vi "ProjetaParabola.vi"(11 "file path (dialog if empty)":path=path "adp.csv") -> (0 "Primeiro":dbl[](array[numeric]), 1 "Ultimo":dbl[](array[numeric]))   [LabVIEW 2019]
uses:
  <vilib>/Analysis/coordinate.llb/3D Coordinate Conversion (Array).vi
  <vilib>/Analysis/_algsub.llb/Real Vector Norm.vi
  <vilib>/Utility/file.llb/Read Delimited Spreadsheet (DBL).vi
  <vilib>/Analysis/polynomials.llb/Polynomial Roots (DBL).vi
  <vilib>/Analysis/NI_AALPro.lvlib
  <vilib>/Analysis/NI_AAL_Geometry.lvlib
panel:
  out "chegada":dbl[](array[numeric])
  out "partida":dbl[](array[numeric])
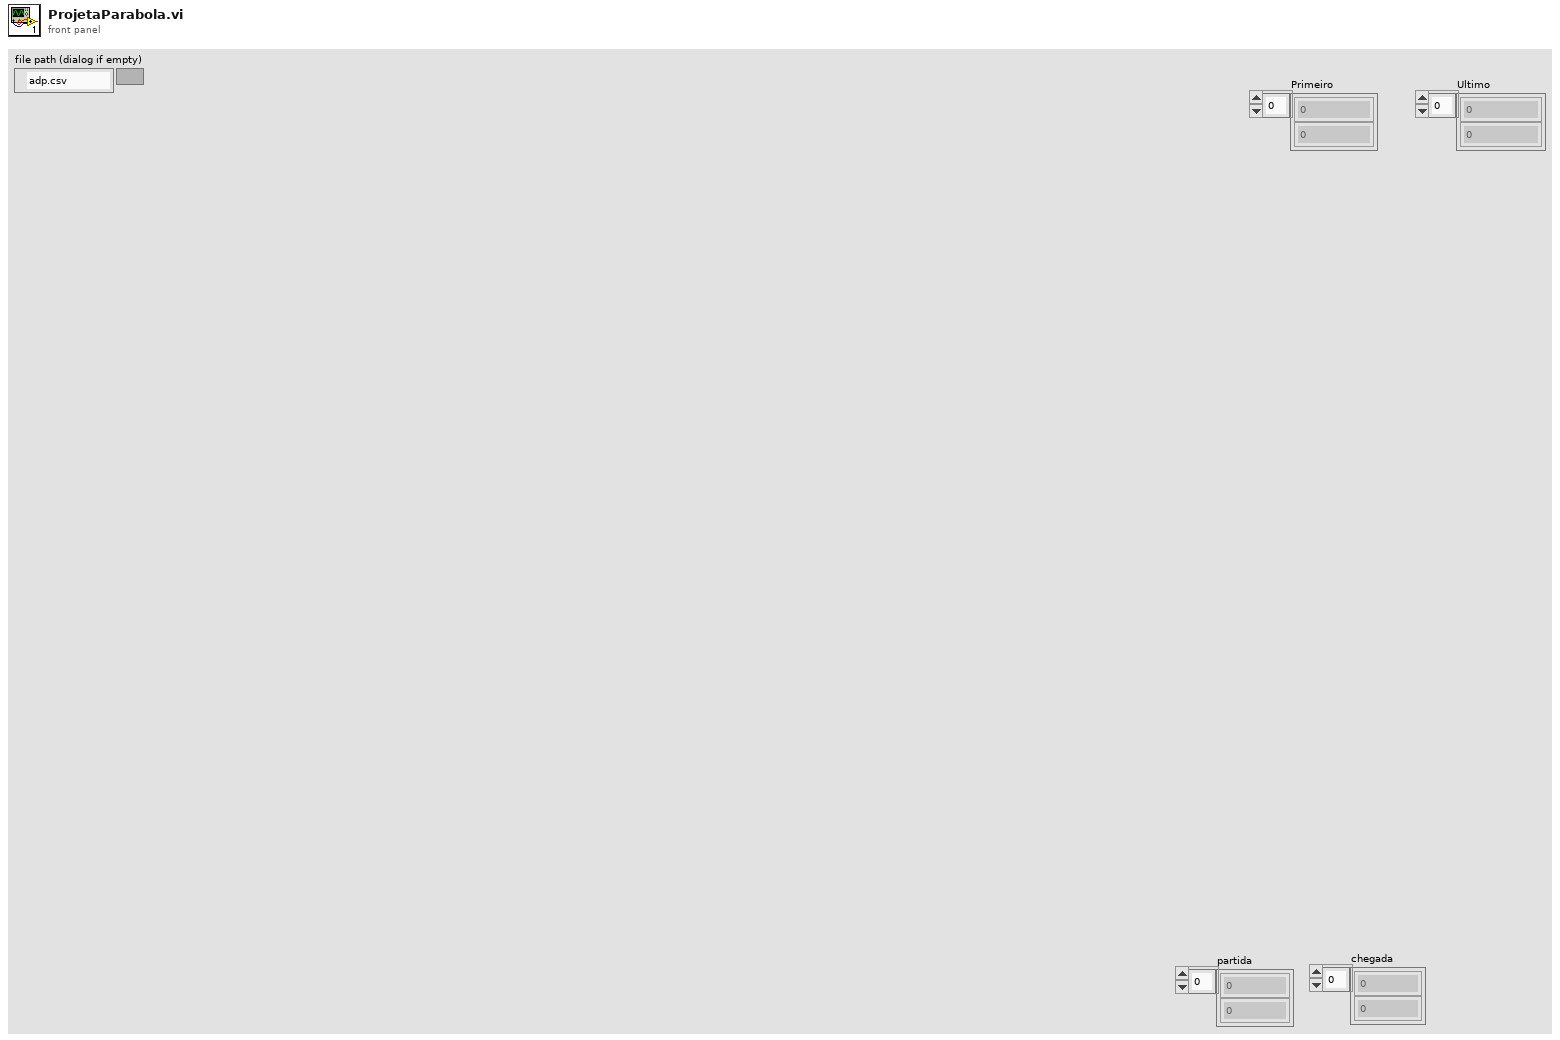
[diagram p1: front panel]
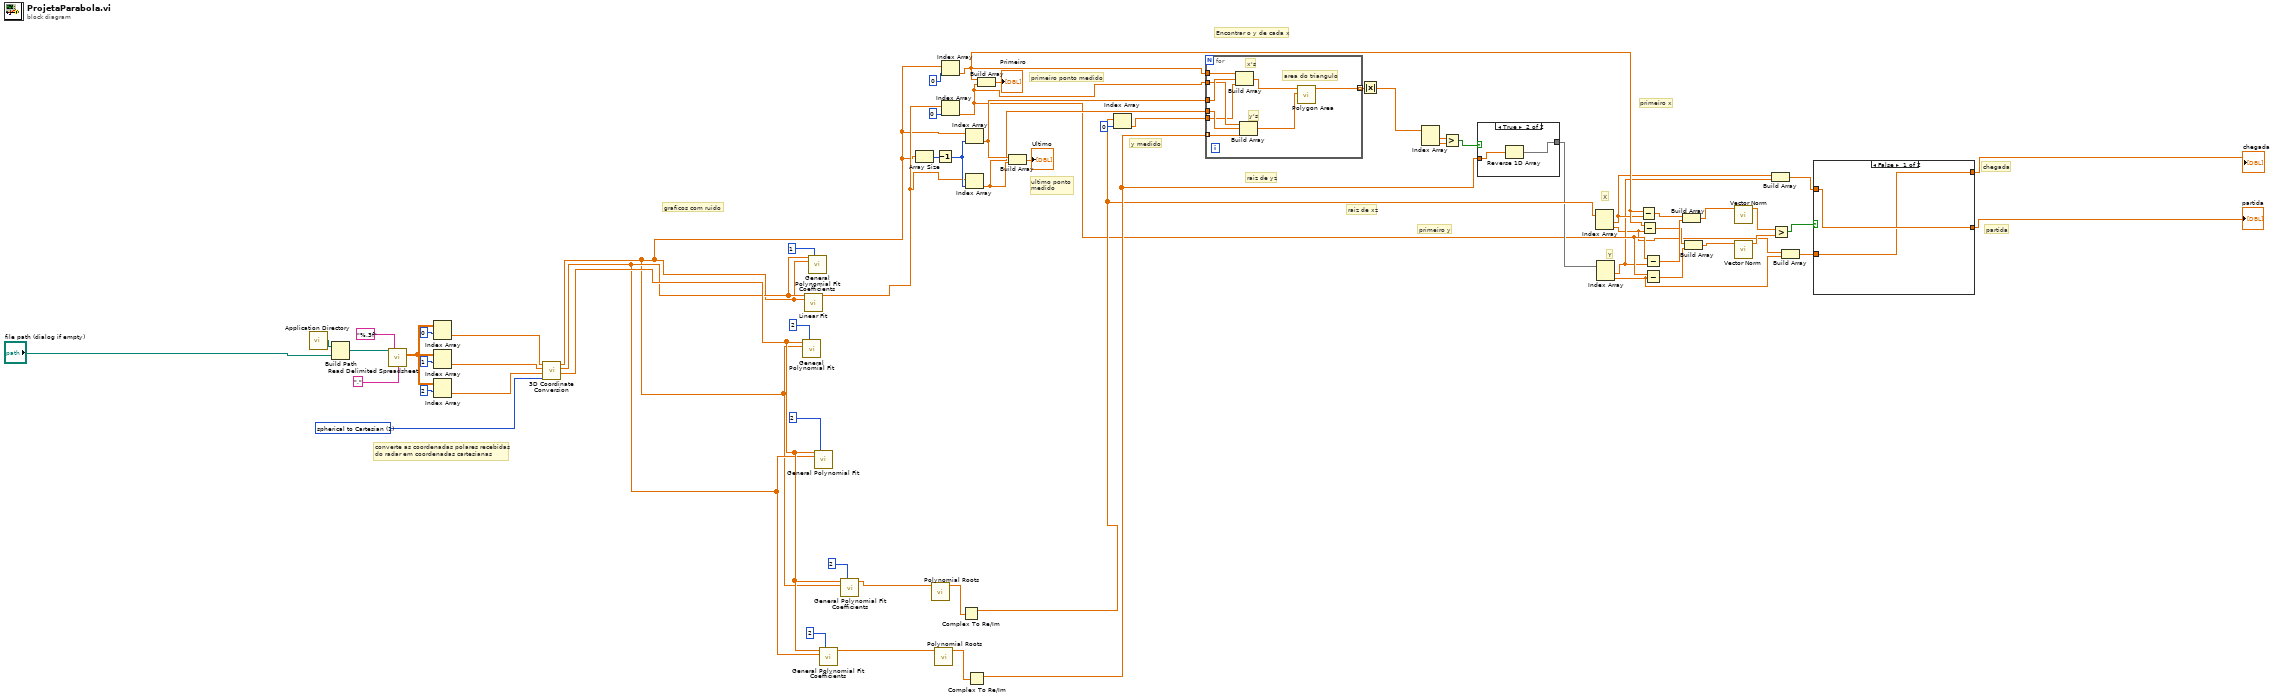
[diagram p0: block diagram]
diagram:
  w58 = u16 1 items=["Cartesian to spherical", "spherical to Cartesian", "Cartesian to cylindrical", "cylindrical to Cartesian", "spherical to cylindrical", "cylindrical to spherical"] ("conversion type")
  # "raiz de yz"
  # "raiz de xz"
  # "primeiro y"
  # "primeiro x"
  # "y medido"
  # "graficos com ruido"
  # "converte as coordenadas polares recebidas \ndo radar em coordenadas cartesianas"
  # "primeiro ponto medido"
  # "ultimo ponto\nmedido"
  # "Encontrar o y de cada x"
  # "partida"
  # "chegada"
  # "Y"
  # "X"
  n1 = call <vilib>:"Application Directory.vi"() -> ("Application Directory"=w56:path)
  n2 = Build Path(base path=w56, name or relative path="file path (dialog if empty)") -> (appended path=w57:path)
  n3 = call-poly <vilib>:"Read Delimited Spreadsheet.vi"("file path (dialog if empty)"=w57, "format (%.3f)"="%.3f", "delimiter (\\t)"="," ("delimiter (\\t)")) -> ("all rows"=w50:dbl[][])  [unwired: 7 in, 5 out]
  n4 = Index Array(array=w50, index (row)=0) -> (element=w46:dbl[])  [unwired: 1 in]
  n5 = Index Array(array=w50, index (row)=1) -> (element=w47:dbl[])  [unwired: 1 in]
  n6 = Index Array(array=w50, index (row)=2) -> (element=w48:dbl[])  [unwired: 1 in]
  n7 = call-poly <vilib>:"3D Coordinate Conversion.vi"("conversion type"=w58, "Axis 3"=w48, "Axis 2"=w47, "Axis 1"=w46) -> ("Axis 3 Out"=w49:dbl[], "Axis 2 Out"=w7:dbl[], "Axis 1 Out"=w1:dbl[])  [unwired: 4 in, 1 out]
  n8 = call <vilib>:"General Polynomial Fit.vi"("Y"=w49, "polynomial order"=2, "X"=w1) -> ()  [unwired: 9 in, 4 out]
  n9 = call <vilib>:"Linear Fit.vi"("Y"=w7, "X"=w1) -> ("Best Linear Fit"=w2:dbl[])  [unwired: 9 in, 4 out]
  n10 = call <vilib>:"General Polynomial Fit Coefficients.vi"("Y"=w7, "polynomial order"=1, "X"=w1) -> ()  [unwired: 11 in, 2 out]
  n11 = call <vilib>:"General Polynomial Fit.vi"("Y"=w49, "polynomial order"=2, "X"=w7) -> ()  [unwired: 9 in, 4 out]
  n12 = call <vilib>:"General Polynomial Fit Coefficients.vi"("Y"=w49, "polynomial order"=2, "X"=w7) -> ("Polynomial Coefficients"=w59:dbl[])  [unwired: 11 in, 1 out]
  n13 = call <vilib>:"General Polynomial Fit Coefficients.vi"("Y"=w49, "polynomial order"=2, "X"=w1) -> ("Polynomial Coefficients"=w12:dbl[])  [unwired: 11 in, 1 out]
  n14 = Array Size(array=w1) -> (size(s)=w41:i32)
  n15 = call-poly <vilib>:"Polynomial Roots.vi"("P(x)"=w12) -> ("Roots"=w39:cdb[])  [unwired: 9 in, 1 out]
  n16 = call-poly <vilib>:"Polynomial Roots.vi"("P(x)"=w59) -> ("Roots"=w38:cdb[])  [unwired: 9 in, 1 out]
  n17 = Decrement(x=w41) -> (x-1=w40:i32)
  n18 = Index Array(array=w2, index=0) -> (element=w26:dbl)
  n19 = Index Array(array=w1, index=0) -> (element=w27:dbl)
  n20 = Complex To Re/Im(x + iy=w39) -> (x=w29:dbl[])  [unwired: 1 out]
  n21 = Index Array(array=w1, index=w40) -> (element=w37:dbl)
  n22 = Index Array(array=w2, index=w40) -> (element=w36:dbl)
  n23 = Complex To Re/Im(x + iy=w38) -> (x=w30:dbl[])  [unwired: 1 out]
  n24 = Build Array(w27, w26) -> (→"Primeiro":dbl[])
  n25 = Build Array(w37, w36) -> (→"Ultimo":dbl[])
  n26 = Index Array(array=w29, index=0) -> (element=w34:dbl)
  n27 = for {
    tunnel: w30 -> [w68] mode=indexing
    tunnel: w27 -> [w72]
    tunnel: w26 -> [w70]
    tunnel: w37 -> [w71]
    tunnel: w36 -> [w69]
    tunnel: [w65] -> w5 mode=indexing
    tunnel: w34 -> [w64]
    # "area do triangulo"
    # "x's"
    # "y's"
    n28 = Build Array(w72, w71, w64) -> (w66:dbl[])
    n29 = Build Array(w70, w69, w68) -> (w67:dbl[])
    n30 = call <vilib>:"Polygon Area.vi"("Y"=w67, "X"=w66) -> ("signed area"=w65:dbl)  [unwired: 8 in, 1 out]
  }
  n31 = Absolute Value(x=w5) -> (abs(x)=w4:dbl[])
  n32 = Index Array(array=w4) -> (element #1=w32:dbl, element #2=w33:dbl)  [unwired: 2 in]
  n33 = Greater?(x=w32, y=w33) -> (0:w31:bool)
  n34 = case shown="True" w31 {
    tunnel: w30 -> [w73 w75]
    tunnel: [w73 w74] -> w28
    frame False {
    }
    frame True {
      n35 = Reverse 1D Array(array=w75) -> (reversed array=w74:dbl[])
    }
  }
  n36 = Index Array(array=w29) -> (element #1=w16:dbl, element #2=w14:dbl)  [unwired: 2 in]
  n37 = Index Array(array=w28) -> (element #1=w15:dbl, element #2=w13:dbl)  [unwired: 2 in]
  n38 = Subtract(x=w27, y=w16) -> (x-y=w25:dbl)
  n39 = Subtract(x=w27, y=w14) -> (x-y=w23:dbl)
  n40 = Subtract(x=w26, y=w15) -> (x-y=w24:dbl)
  n41 = Subtract(x=w26, y=w13) -> (x-y=w22:dbl)
  n42 = Build Array(w25, w24) -> (w18:dbl[])
  n43 = Build Array(w23, w22) -> (w17:dbl[])
  n44 = call-poly <vilib>:"Vector Norm.vi"("Input Vector"=w17) -> ("norm"=w20:dbl)  [unwired: 9 in, 1 out]
  n45 = call-poly <vilib>:"Vector Norm.vi"("Input Vector"=w18) -> ("norm"=w21:dbl)  [unwired: 9 in, 1 out]
  n46 = Build Array(w16, w15) -> (w10:dbl[])
  n47 = Greater?(x=w21, y=w20) -> (0:w19:bool)
  n48 = Build Array(w14, w13) -> (w11:dbl[])
  n49 = case shown="False" w19 {
    tunnel: [w77 w79] -> w9
    tunnel: w11 -> [w76 w79]
    tunnel: w10 -> [w77 w78]
    tunnel: [w76 w78] -> w8
    frame False {
    }
    frame True {
    }
  }
  "partida" <- w9
  "chegada" <- w8
